vi "Get Chamber Status.vi"(8 "error in (no error)":errorcluster, 9 "Time Interval (ms)":u32) -> (0 "error out":errorcluster, 1 "Ramp Rate (deg C / second)":dbl, 2 "Temperature Set Point (deg C)":dbl, 3 "Actual Temperature":dbl, 4 "Application Exit":bool, 6 "Heater State":bool)   [LabVIEW 2015, in "Thermal Chamber Response Simulator.lvlib"]
doc: "Get the status of the chamber from the AE.\n____\nDelacor QMH Thermal Chamber Examples 4.0.0.21\nCopyright (c) 2018, Delacor"
uses:
  Thermal Chamber Response Simulator.lvlib
  Action--enum.ctl
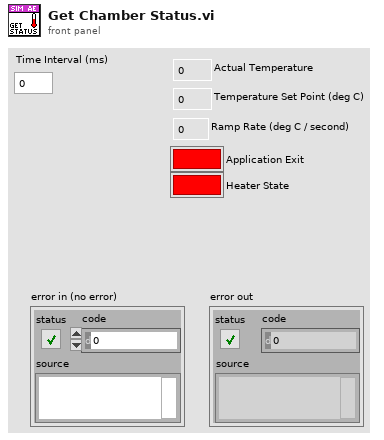
[diagram p1: front panel]
types:
  T1 = typedef "Thermal Chamber Response Simulator.lvlib/Action--enum.ctl" = enum16{"Initialize", "Set Temperature Required", "Set Ramp Rate", "Get Status", "Disable Heater", "Enable Heater", "Exit Application"}
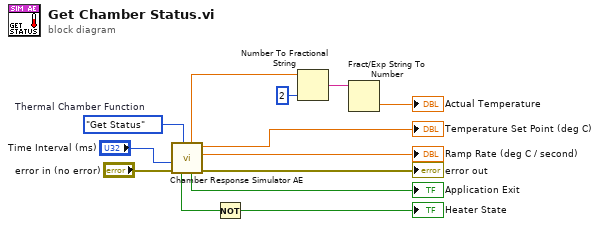
[diagram p0: block diagram]
diagram:
  w4 = Action--enum."Get Status"  # Thermal Chamber Function
  n1 = call "Chamber Response Simulator AE.vi"("Thermal Chamber Function"=w4, "error in (no error)"="error in (no error)", "Time Interval (ms)"="Time Interval (ms)") -> ("error out"=→"error out":errorcluster, "Ramp Rate out"=→"Ramp Rate (deg C / second)":dbl, "Temperature Set Point out"=→"Temperature Set Point (deg C)":dbl, "Application Exit"=→"Application Exit":bool, "Actual Temperature"=w3:dbl, "Shutdown Furnace?"=w11:bool)  [unwired: 3 in]
  n2 = Not(x=w11) -> (.not. x?=→"Heater State":bool)
  n3 = Number To Fractional String(number=w3, precision (6)=i16 2) -> (F-format string=w7:string)  [unwired: 2 in]
  n4 = Fract/Exp String To Number(string=w7) -> (number=→"Actual Temperature":dbl)  [unwired: 3 in, 1 out]
